vi "test TCX read (installed 71).vi"() -> ()   [LabVIEW 2011] (continued)
9</AltitudeMeters><DistanceMeters>17425.164</DistanceMeters><Cadence>84</Cadence><Extensions><TPX xmlns=\"http://www.garmin.com/xmlschemas/ActivityExtension/v2\"><Watts>247</Watts></TPX></Extensions></Trackpoint><Trackpoint><Time>2008-03-03T23:16:37Z</Time><Position><LatitudeDegrees>35.875664</LatitudeDegrees><LongitudeDegrees>-78.918461</LongitudeDegrees></Position><AltitudeMeters>60.220</AltitudeMeters><DistanceMeters>17434.398</DistanceMeters><Cadence>84</Cadence><Extensions><TPX xmlns=\"http://www.garmin.com/xmlschemas/ActivityExtension/v2\"><Watts>257</Watts></TPX></Extensions></Trackpoint><Trackpoint><Time>2008-03-03T23:16:38Z</Time><Position><LatitudeDegrees>35.875658</LatitudeDegrees><LongitudeDegrees>-78.918560</LongitudeDegrees></Position><AltitudeMeters>60.220</AltitudeMeters><DistanceMeters>17443.352</DistanceMeters><Cadence>83</Cadence><Extensions><TPX xmlns=\"http://www.garmin.com/xmlschemas/ActivityExtension/v2\"><Watts>228</Watts></TPX></Extensions></Trackpoint><Trackpoint><Time>2008-03-03T23:16:39Z</Time><Position><LatitudeDegrees>35.875651</LatitudeDegrees><LongitudeDegrees>-78.918658</LongitudeDegrees></Position><AltitudeMeters>60.220</AltitudeMeters><DistanceMeters>17452.232</DistanceMeters><Cadence>83</Cadence><Extensions><TPX xmlns=\"http://www.garmin.com/xmlschemas/ActivityExtension/v2\"><Watts>229</Watts></TPX></Extensions></Trackpoint><Trackpoint><Time>2008-03-03T23:16:40Z</Time><Position><LatitudeDegrees>35.875641</LatitudeDegrees><LongitudeDegrees>-78.918756</LongitudeDegrees></Position><AltitudeMeters>60.220</AltitudeMeters><DistanceMeters>17461.098</DistanceMeters><Cadence>81</Cadence><Extensions><TPX xmlns=\"http://www.garmin.com/xmlschemas/ActivityExtension/v2\"><Watts>206</Watts></TPX></Extensions></Trackpoint><Trackpoint><Time>2008-03-03T23:16:41Z</Time><Position><LatitudeDegrees>35.875632</LatitudeDegrees><LongitudeDegrees>-78.918851</LongitudeDegrees></Position><AltitudeMeters>60.220</AltitudeMeters><DistanceMeters>17469.729</DistanceMeters><Cadence>80</Cadence><Extensions><TPX xmlns=\"http://www.garmin.com/xmlschemas/ActivityExtension/v2\"><Watts>194</Watts></TPX></Extensions></Trackpoint><Trackpoint><Time>2008-03-03T23:16:42Z</Time><Position><LatitudeDegrees>35.875624</LatitudeDegrees><LongitudeDegrees>-78.918945</LongitudeDegrees></Position><AltitudeMeters>60.700</AltitudeMeters><DistanceMeters>17478.252</DistanceMeters><Cadence>77</Cadence><Extensions><TPX xmlns=\"http://www.garmin.com/xmlschemas/ActivityExtension/v2\"><Watts>145</Watts></TPX></Extensions></Trackpoint><Trackpoint><Time>2008-03-03T23:16:43Z</Time><Position><LatitudeDegrees>35.875617</LatitudeDegrees><LongitudeDegrees>-78.919037</LongitudeDegrees></Position><AltitudeMeters>60.220</AltitudeMeters><DistanceMeters>17486.607</DistanceMeters><Cadence>76</Cadence><Extensions><TPX xmlns=\"http://www.garmin.com/xmlschemas/ActivityExtension/v2\"><Watts>140</Watts></TPX></Extensions></Trackpoint><Trackpoint><Time>2008-03-03T23:16:44Z</Time><Position><LatitudeDegrees>35.875609</LatitudeDegrees><LongitudeDegrees>-78.919127</LongitudeDegrees></Position><AltitudeMeters>61.181</AltitudeMeters><DistanceMeters>17494.744</DistanceMeters><Cadence>74</Cadence><Extensions><TPX xmlns=\"http://www.garmin.com/xmlschemas/ActivityExtension/v2\"><Watts>140</Watts></TPX></Extensions></Trackpoint><Trackpoint><Time>2008-03-03T23:16:45Z</Time><Position><LatitudeDegrees>35.875602</LatitudeDegrees><LongitudeDegrees>-78.919214</LongitudeDegrees></Position><AltitudeMeters>61.181</AltitudeMeters><DistanceMeters>17502.676</DistanceMeters><Cadence>73</Cadence><Extensions><TPX xmlns=\"http://www.garmin.com/xmlschemas/ActivityExtension/v2\"><Watts>144</Watts></TPX></Extensions></Trackpoint><Trackpoint><Time>2008-03-03T23:16:46Z</Time><Position><LatitudeDegrees>35.875596</LatitudeDegrees><LongitudeDegrees>-78.919299</LongitudeDegrees></Position><AltitudeMeters>61.662</AltitudeMeters><DistanceMeters>17510.342</DistanceMeters><Cadence>71</Cadence><Extensions><TPX xmlns=\"http://www.garmin.com/xmlschemas/ActivityExtension/v2\"><Watts>160</Watts></TPX></Extensions></Trackpoint><Trackpoint><Time>2008-03-03T23:16:47Z</Time><Position><LatitudeDegrees>35.875590</LatitudeDegrees><LongitudeDegrees>-78.919382</LongitudeDegrees></Position><AltitudeMeters>61.181</AltitudeMeters><DistanceMeters>17517.861</DistanceMeters><Cadence>68</Cadence><Extensions><TPX xmlns=\"http://www.garmin.com/xmlschemas/ActivityExtension/v2\"><Watts>179</Watts></TPX></Extensions></Trackpoint><Trackpoint><Time>2008-03-03T23:16:48Z</Time><Position><LatitudeDegrees>35.875584</LatitudeDegrees><LongitudeDegrees>-78.919463</LongitudeDegrees></Position><AltitudeMeters>61.662</AltitudeMeters><DistanceMeters>17525.182</DistanceMeters><Cadence>67</Cadence><Extensions><TPX xmlns=\"http://www.garmin.com/xmlschemas/ActivityExtension/v2\"><Watts>190</Watts></TPX></Extensions></Trackpoint><Trackpoint><Time>2008-03-03T23:16:49Z</Time><Position><LatitudeDegrees>35.875578</LatitudeDegrees><LongitudeDegrees>-78.919542</LongitudeDegrees></Position><AltitudeMeters>61.662</AltitudeMeters><DistanceMeters>17532.338</DistanceMeters><Cadence>67</Cadence><Extensions><TPX xmlns=\"http://www.garmin.com/xmlschemas/ActivityExtension/v2\"><Watts>189</Watts></TPX></Extensions></Trackpoint><Trackpoint><Time>2008-03-03T23:16:50Z</Time><Position><LatitudeDegrees>35.875573</LatitudeDegrees><LongitudeDegrees>-78.919619</LongitudeDegrees></Position><AltitudeMeters>62.142</AltitudeMeters><DistanceMeters>17539.316</DistanceMeters><Cadence>65</Cadence><Extensions><TPX xmlns=\"http://www.garmin.com/xmlschemas/ActivityExtension/v2\"><Watts>213</Watts></TPX></Extensions></Trackpoint><Trackpoint><Time>2008-03-03T23:16:51Z</Time><Position><LatitudeDegrees>35.875567</LatitudeDegrees><LongitudeDegrees>-78.919694</LongitudeDegrees></Position><AltitudeMeters>62.142</AltitudeMeters><DistanceMeters>17546.102</DistanceMeters><Cadence>65</Cadence><Extensions><TPX xmlns=\"http://www.garmin.com/xmlschemas/ActivityExtension/v2\"><Watts>212</Watts></TPX></Extensions></Trackpoint><Trackpoint><Time>2008-03-03T23:16:52Z</Time><Position><LatitudeDegrees>35.875561</LatitudeDegrees><LongitudeDegrees>-78.919766</LongitudeDegrees></Position><AltitudeMeters>62.623</AltitudeMeters><DistanceMeters>17552.578</DistanceMeters><Cadence>67</Cadence><Extensions><TPX xmlns=\"http://www.garmin.com/xmlschemas/ActivityExtension/v2\"><Watts>211</Watts></TPX></Extensions></Trackpoint><Trackpoint><Time>2008-03-03T23:16:53Z</Time><Position><LatitudeDegrees>35.875555</LatitudeDegrees><LongitudeDegrees>-78.919835</LongitudeDegrees></Position><AltitudeMeters>62.623</AltitudeMeters><DistanceMeters>17558.822</DistanceMeters><Cadence>64</Cadence><Extensions><TPX xmlns=\"http://www.garmin.com/xmlschemas/ActivityExtension/v2\"><Watts>225</Watts></TPX></Extensions></Trackpoint><Trackpoint><Time>2008-03-03T23:16:54Z</Time><Position><LatitudeDegrees>35.875549</LatitudeDegrees><LongitudeDegrees>-78.919905</LongitudeDegrees></Position><AltitudeMeters>62.623</AltitudeMeters><DistanceMeters>17565.227</DistanceMeters><Cadence>66</Cadence><Extensions><TPX xmlns=\"http://www.garmin.com/xmlschemas/ActivityExtension/v2\"><Watts>266</Watts></TPX></Extensions></Trackpoint><Trackpoint><Time>2008-03-03T23:16:55Z</Time><Position><LatitudeDegrees>35.875535</LatitudeDegrees><LongitudeDegrees>-78.919978</LongitudeDegrees></Position><AltitudeMeters>63.104</AltitudeMeters><DistanceMeters>17571.996</DistanceMeters><Cadence>68</Cadence><Extensions><TPX xmlns=\"http://www.garmin.com/xmlschemas/ActivityExtension/v2\"><Watts>407</Watts></TPX></Extensions></Trackpoint><Trackpoint><Time>2008-03-03T23:16:56Z</Time><Position><LatitudeDegrees>35.875527</LatitudeDegrees><LongitudeDegrees>-78.920052</LongitudeDegrees></Position><AltitudeMeters>63.104</AltitudeMeters><DistanceMeters>17578.701</DistanceMeters><Cadence>71</Cadence><Extensions><TPX xmlns=\"http://www.garmin.com/xmlschemas/ActivityExtension/v2\"><Watts>440</Watts></TPX></Extensions></Trackpoint><Trackpoint><Time>2008-03-03T23:16:57Z</Time><Position><LatitudeDegrees>35.875524</LatitudeDegrees><LongitudeDegrees>-78.920126</LongitudeDegrees></Position><AltitudeMeters>63.584</AltitudeMeters><DistanceMeters>17585.479</DistanceMeters><Cadence>73</Cadence><Extensions><TPX xmlns=\"http://www.garmin.com/xmlschemas/ActivityExtension/v2\"><Watts>527</Watts></TPX></Extensions></Trackpoint><Trackpoint><Time>2008-03-03T23:16:58Z</Time><Position><LatitudeDegrees>35.875522</LatitudeDegrees><LongitudeDegrees>-78.920204</LongitudeDegrees></Position><AltitudeMeters>63.584</AltitudeMeters><DistanceMeters>17592.449</DistanceMeters><Cadence>74</Cadence><Extensions><TPX xmlns=\"http://www.garmin.com/xmlschemas/ActivityExtension/v2\"><Watts>618</Watts></TPX></Extensions></Trackpoint><Trackpoint><Time>2008-03-03T23:16:59Z</Time><Position><LatitudeDegrees>35.875519</LatitudeDegrees><LongitudeDegrees>-78.920284</LongitudeDegrees></Position><AltitudeMeters>64.065</AltitudeMeters><DistanceMeters>17599.703</DistanceMeters><Cadence>76</Cadence><Extensions><TPX xmlns=\"http://www.garmin.com/xmlschemas/ActivityExtension/v2\"><Watts>615</Watts></TPX></Extensions></Trackpoint><Trackpoint><Time>2008-03-03T23:17:00Z</Time><Position><LatitudeDegrees>35.875519</LatitudeDegrees><LongitudeDegrees>-78.920364</LongitudeDegrees></Position><AltitudeMeters>64.546</AltitudeMeters><DistanceMeters>17607.000</DistanceMeters><Cadence>76</Cadence><Extensions><TPX xmlns=\"http://www.garmin.com/xmlschemas/ActivityExtension/v2\"><Watts>600</Watts></TPX></Extensions></Trackpoint><Trackpoint><Time>2008-03-03T23:17:01Z</Time><Position><LatitudeDegrees>35.875518</LatitudeDegrees><LongitudeDegrees>-78.920446</LongitudeDegrees></Position><AltitudeMeters>65.507</AltitudeMeters><DistanceMeters>17614.344</DistanceMeters><Cadence>76</Cadence><Extensions><TPX xmlns=\"http://www.garmin.com/xmlschemas/ActivityExtension/v2\"><Watts>605</Watts></TPX></Extensions></Trackpoint><Trackpoint><Time>2008-03-03T23:17:02Z</Time><Position><LatitudeDegrees>35.875515</LatitudeDegrees><LongitudeDegrees>-78.920525</LongitudeDegrees></Position><AltitudeMeters>65.988</AltitudeMeters><DistanceMeters>17621.482</DistanceMeters><Cadence>73</Cadence><Extensions><TPX xmlns=\"http://www.garmin.com/xmlschemas/ActivityExtension/v2\"><Watts>509</Watts></TPX></Extensions></Trackpoint><Trackpoint><Time>2008-03-03T23:17:03Z</Time><Position><LatitudeDegrees>35.875514</LatitudeDegrees><LongitudeDegrees>-78.920601</LongitudeDegrees></Position><AltitudeMeters>66.468</AltitudeMeters><DistanceMeters>17628.330</DistanceMeters><Cadence>72</Cadence><Extensions><TPX xmlns=\"http://www.garmin.com/xmlschemas/ActivityExtension/v2\"><Watts>498</Watts></TPX></Extensions></Trackpoint><Trackpoint><Time>2008-03-03T23:17:04Z</Time><Position><LatitudeDegrees>35.875514</LatitudeDegrees><LongitudeDegrees>-78.920677</LongitudeDegrees></Position><AltitudeMeters>66.468</AltitudeMeters><DistanceMeters>17635.150</DistanceMeters><Cadence>71</Cadence><Extensions><TPX xmlns=\"http://www.garmin.com/xmlschemas/ActivityExtension/v2\"><Watts>409</Watts></TPX></Extensions></Trackpoint><Trackpoint><Time>2008-03-03T23:17:05Z</Time><Position><LatitudeDegrees>35.875514</LatitudeDegrees><LongitudeDegrees>-78.920753</LongitudeDegrees></Position><AltitudeMeters>66.468</AltitudeMeters><DistanceMeters>17642.037</DistanceMeters><Cadence>72</Cadence><Extensions><TPX xmlns=\"http://www.garmin.com/xmlschemas/ActivityExtension/v2\"><Watts>369</Watts></TPX></Extensions></Trackpoint><Trackpoint><Time>2008-03-03T23:17:06Z</Time><Position><LatitudeDegrees>35.875510</LatitudeDegrees><LongitudeDegrees>-78.920830</LongitudeDegrees></Position><AltitudeMeters>66.949</AltitudeMeters><DistanceMeters>17649.055</DistanceMeters><Cadence>73</Cadence><Extensions><TPX xmlns=\"http://www.garmin.com/xmlschemas/ActivityExtension/v2\"><Watts>334</Watts></TPX></Extensions></Trackpoint><Trackpoint><Time>2008-03-03T23:17:07Z</Time><Position><LatitudeDegrees>35.875506</LatitudeDegrees><LongitudeDegrees>-78.920910</LongitudeDegrees></Position><AltitudeMeters>67.430</AltitudeMeters><DistanceMeters>17656.324</DistanceMeters><Cadence>75</Cadence><Extensions><TPX xmlns=\"http://www.garmin.com/xmlschemas/ActivityExtension/v2\"><Watts>331</Watts></TPX></Extensions></Trackpoint><Trackpoint><Time>2008-03-03T23:17:08Z</Time><Position><LatitudeDegrees>35.875502</LatitudeDegrees><LongitudeDegrees>-78.920993</LongitudeDegrees></Position><AltitudeMeters>67.910</AltitudeMeters><DistanceMeters>17663.768</DistanceMeters><Cadence>79</Cadence><Extensions><TPX xmlns=\"http://www.garmin.com/xmlschemas/ActivityExtension/v2\"><Watts>322</Watts></TPX></Extensions></Trackpoint><Trackpoint><Time>2008-03-03T23:17:09Z</Time><Position><LatitudeDegrees>35.875499</LatitudeDegrees><LongitudeDegrees>-78.921077</LongitudeDegrees></Position><AltitudeMeters>67.430</AltitudeMeters><DistanceMeters>17671.379</DistanceMeters><Cadence>78</Cadence><Extensions><TPX xmlns=\"http://www.garmin.com/xmlschemas/ActivityExtension/v2\"><Watts>318</Watts></TPX></Extensions></Trackpoint><Trackpoint><Time>2008-03-03T23:17:10Z</Time><Position><LatitudeDegrees>35.875497</LatitudeDegrees><LongitudeDegrees>-78.921161</LongitudeDegrees></Position><AltitudeMeters>67.430</AltitudeMeters><DistanceMeters>17679.006</DistanceMeters><Cadence>78</Cadence><Extensions><TPX xmlns=\"http://www.garmin.com/xmlschemas/ActivityExtension/v2\"><Watts>224</Watts></TPX></Extensions></Trackpoint><Trackpoint><Time>2008-03-03T23:17:11Z</Time><Position><LatitudeDegrees>35.875497</LatitudeDegrees><LongitudeDegrees>-78.921246</LongitudeDegrees></Position><AltitudeMeters>67.430</AltitudeMeters><DistanceMeters>17686.682</DistanceMeters><Cadence>79</Cadence><Extensions><TPX xmlns=\"http://www.garmin.com/xmlschemas/ActivityExtension/v2\"><Watts>133</Watts></TPX></Extensions></Trackpoint><Trackpoint><Time>2008-03-03T23:17:12Z</Time><Position><LatitudeDegrees>35.875498</LatitudeDegrees><LongitudeDegrees>-78.921332</LongitudeDegrees></Position><AltitudeMeters>67.910</AltitudeMeters><DistanceMeters>17694.391</DistanceMeters><Cadence>79</Cadence><Extensions><TPX xmlns=\"http://www.garmin.com/xmlschemas/ActivityExtension/v2\"><Watts>116</Watts></TPX></Extensions></Trackpoint><Trackpoint><Time>2008-03-03T23:17:13Z</Time><Position><LatitudeDegrees>35.875497</LatitudeDegrees><LongitudeDegrees>-78.921417</LongitudeDegrees></Position><AltitudeMeters>67.910</AltitudeMeters><DistanceMeters>17702.156</DistanceMeters><Cadence>79</Cadence><Extensions><TPX xmlns=\"http://www.garmin.com/xmlschemas/ActivityExtension/v2\"><Watts>105</Watts></TPX></Extensions></Trackpoint><Trackpoint><Time>2008-03-03T23:17:14Z</Time><Position><LatitudeDegrees>35.875496</LatitudeDegrees><LongitudeDegrees>-78.921503</LongitudeDegrees></Position><AltitudeMeters>67.910</AltitudeMeters><DistanceMeters>17709.824</DistanceMeters><Cadence>79</Cadence><Extensions><TPX xmlns=\"http://www.garmin.com/xmlschemas/ActivityExtension/v2\"><Watts>101</Watts></TPX></Extensions></Trackpoint><Trackpoint><Time>2008-03-03T23:17:15Z</Time><Position><LatitudeDegrees>35.875492</LatitudeDegrees><LongitudeDegrees>-78.921586</LongitudeDegrees></Position><AltitudeMeters>67.910</AltitudeMeters><DistanceMeters>17717.307</DistanceMeters><Cadence>77</Cadence><Extensions><TPX xmlns=\"http://www.garmin.com/xmlschemas/ActivityExtension/v2\"><Watts>104</Watts></TPX></Extensions></Trackpoint><Trackpoint><Time>2008-03-03T23:17:16Z</Time><Position><LatitudeDegrees>35.875488</LatitudeDegrees><LongitudeDegrees>-78.921667</LongitudeDegrees></Position><AltitudeMeters>67.910</AltitudeMeters><DistanceMeters>17724.688</DistanceMeters><Cadence>77</Cadence><Extensions><TPX xmlns=\"http://www.garmin.com/xmlschemas/ActivityExtension/v2\"><Watts>103</Watts></TPX></Extensions></Trackpoint><Trackpoint><Time>2008-03-03T23:17:17Z</Time><Position><LatitudeDegrees>35.875483</LatitudeDegrees><LongitudeDegrees>-78.921747</LongitudeDegrees></Position><AltitudeMeters>67.910</AltitudeMeters><DistanceMeters>17731.865</DistanceMeters><Cadence>73</Cadence><Extensions><TPX xmlns=\"http://www.garmin.com/xmlschemas/ActivityExtension/v2\"><Watts>125</Watts></TPX></Extensions></Trackpoint><Trackpoint><Time>2008-03-03T23:17:18Z</Time><Position><LatitudeDegrees>35.875477</LatitudeDegrees><LongitudeDegrees>-78.921826</LongitudeDegrees></Position><AltitudeMeters>67.910</AltitudeMeters><DistanceMeters>17739.020</DistanceMeters><Cadence>75</Cadence><Extensions><TPX xmlns=\"http://www.garmin.com/xmlschemas/ActivityExtension/v2\"><Watts>187</Watts></TPX></Extensions></Trackpoint><Trackpoint><Time>2008-03-03T23:17:19Z</Time><Position><LatitudeDegrees>35.875471</LatitudeDegrees><LongitudeDegrees>-78.921905</LongitudeDegrees></Position><AltitudeMeters>68.391</AltitudeMeters><DistanceMeters>17746.203</DistanceMeters><Cadence>75</Cadence><Extensions><TPX xmlns=\"http://www.garmin.com/xmlschemas/ActivityExtension/v2\"><Watts>304</Watts></TPX></Extensions></Trackpoint><Trackpoint><Time>2008-03-03T23:17:20Z</Time><Position><LatitudeDegrees>35.875465</LatitudeDegrees><LongitudeDegrees>-78.921982</LongitudeDegrees></Position><AltitudeMeters>68.872</AltitudeMeters><DistanceMeters>17753.166</DistanceMeters><Cadence>73</Cadence><Extensions><TPX xmlns=\"http://www.garmin.com/xmlschemas/ActivityExtension/v2\"><Watts>365</Watts></TPX></Extensions></Trackpoint><Trackpoint><Time>2008-03-03T23:17:21Z</Time><Position><LatitudeDegrees>35.875460</LatitudeDegrees><LongitudeDegrees>-78.922058</LongitudeDegrees></Position><AltitudeMeters>68.872</AltitudeMeters><DistanceMeters>17760.088</DistanceMeters><Cadence>73</Cadence><Extensions><TPX xmlns=\"http://www.garmin.com/xmlschemas/ActivityExtension/v2\"><Watts>361</Watts></TPX></Extensions></Trackpoint><Trackpoint><Time>2008-03-03T23:17:22Z</Time><Position><LatitudeDegrees>35.875456</LatitudeDegrees><LongitudeDegrees>-78.922133</LongitudeDegrees></Position><AltitudeMeters>69.352</AltitudeMeters><DistanceMeters>17766.865</DistanceMeters><Cadence>70</Cadence><Extensions><TPX xmlns=\"http://www.garmin.com/xmlschemas/ActivityExtension/v2\"><Watts>317</Watts></TPX></Extensions></Trackpoint><Trackpoint><Time>2008-03-03T23:17:23Z</Time><Position><LatitudeDegrees>35.875451</LatitudeDegrees><LongitudeDegrees>-78.922207</LongitudeDegrees></Position><AltitudeMeters>69.833</AltitudeMeters><DistanceMeters>17773.584</DistanceMeters><Cadence>70</Cadence><Extensions><TPX xmlns=\"http://www.garmin.com/xmlschemas/ActivityExtension/v2\"><Watts>340</Watts></TPX></Extensions></Trackpoint><Trackpoint><Time>2008-03-03T23:17:24Z</Time><Position><LatitudeDegrees>35.875446</LatitudeDegrees><LongitudeDegrees>-78.922283</LongitudeDegrees></Position><AltitudeMeters>69.833</AltitudeMeters><DistanceMeters>17780.492</DistanceMeters><Cadence>75</Cadence><Extensions><TPX xmlns=\"http://www.garmin.com/xmlschemas/ActivityExtension/v2\"><Watts>332</Watts></TPX></Extensions></Trackpoint><Trackpoint><Time>2008-03-03T23:17:25Z</Time><Position><LatitudeDegrees>35.875445</LatitudeDegrees><LongitudeDegrees>-78.922363</LongitudeDegrees></Position><AltitudeMeters>70.313</AltitudeMeters><DistanceMeters>17787.660</DistanceMeters><Cadence>73</Cadence><Extensions><TPX xmlns=\"http://www.garmin.com/xmlschemas/ActivityExtension/v2\"><Watts>305</Watts></TPX></Extensions></Trackpoint><Trackpoint><Time>2008-03-03T23:17:26Z</Time><Position><LatitudeDegrees>35.875444</LatitudeDegrees><LongitudeDegrees>-78.922441</LongitudeDegrees></Position><AltitudeMeters>70.313</AltitudeMeters><DistanceMeters>17794.773</DistanceMeters><Cadence>73</Cadence><Extensions><TPX xmlns=\"http://www.garmin.com/xmlschemas/ActivityExtension/v2\"><Watts>224</Watts></TPX></Extensions></Trackpoint><Trackpoint><Time>2008-03-03T23:17:27Z</Time><Position><LatitudeDegrees>35.875442</LatitudeDegrees><LongitudeDegrees>-78.922520</LongitudeDegrees></Position><AltitudeMeters>70.313</AltitudeMeters><DistanceMeters>17801.924</DistanceMeters><Cadence>74</Cadence><Extensions><TPX xmlns=\"http://www.garmin.com/xmlschemas/ActivityExtension/v2\"><Watts>148</Watts></TPX></Extensions></Trackpoint><Trackpoint><Time>2008-03-03T23:17:28Z</Time><Position><LatitudeDegrees>35.875442</LatitudeDegrees><LongitudeDegrees>-78.922601</LongitudeDegrees></Position><AltitudeMeters>70.313</AltitudeMeters><DistanceMeters>17809.150</DistanceMeters><Cadence>74</Cadence><Extensions><TPX xmlns=\"http://www.garmin.com/xmlschemas/ActivityExtension/v2\"><Watts>122</Watts></TPX></Extensions></Trackpoint><Trackpoint><Time>2008-03-03T23:17:29Z</Time><Position><LatitudeDegrees>35.875442</LatitudeDegrees><LongitudeDegrees>-78.922683</LongitudeDegrees></Position><AltitudeMeters>70.794</AltitudeMeters><DistanceMeters>17816.596</DistanceMeters><Cadence>77</Cadence><Extensions><TPX xmlns=\"http://www.garmin.com/xmlschemas/ActivityExtension/v2\"><Watts>92</Watts></TPX></Extensions></Trackpoint><Trackpoint><Time>2008-03-03T23:17:30Z</Time><Position><LatitudeDegrees>35.875443</LatitudeDegrees><LongitudeDegrees>-78.922767</LongitudeDegrees></Position><AltitudeMeters>69.833</AltitudeMeters><DistanceMeters>17824.229</DistanceMeters><Cadence>79</Cadence><Extensions><TPX xmlns=\"http://www.garmin.com/xmlschemas/ActivityExtension/v2\"><Watts>79</Watts></TPX></Extensions></Trackpoint><Trackpoint><Time>2008-03-03T23:17:31Z</Time><Position><LatitudeDegrees>35.875442</LatitudeDegrees><LongitudeDegrees>-78.922856</LongitudeDegrees></Position><AltitudeMeters>69.833</AltitudeMeters><DistanceMeters>17832.281</DistanceMeters><Cadence>68</Cadence><Extensions><TPX xmlns=\"http://www.garmin.com/xmlschemas/ActivityExtension/v2\"><Watts>70</Watts></TPX></Extensions></Trackpoint><Trackpoint><Time>2008-03-03T23:17:32Z</Time><Position><LatitudeDegrees>35.875442</LatitudeDegrees><LongitudeDegrees>-78.922951</LongitudeDegrees></Position><AltitudeMeters>69.352</AltitudeMeters><DistanceMeters>17840.867</DistanceMeters><Cadence>69</Cadence><Extensions><TPX xmlns=\"http://www.garmin.com/xmlschemas/ActivityExtension/v2\"><Watts>69</Watts></TPX></Extensions></Trackpoint><Trackpoint><Time>2008-03-03T23:17:33Z</Time><Position><LatitudeDegrees>35.875442</LatitudeDegrees><LongitudeDegrees>-78.923052</LongitudeDegrees></Position><AltitudeMeters>69.352</AltitudeMeters><DistanceMeters>17850.025</DistanceMeters><Cadence>73</Cadence><Extensions><TPX xmlns=\"http://www.garmin.com/xmlschemas/ActivityExtension/v2\"><Watts>69</Watts></TPX></Extensions></Trackpoint><Trackpoint><Time>2008-03-03T23:17:34Z</Time><Position><LatitudeDegrees>35.875441</LatitudeDegrees><LongitudeDegrees>-78.923158</LongitudeDegrees></Position><AltitudeMeters>68.872</AltitudeMeters><DistanceMeters>17859.643</DistanceMeters><Cadence>78</Cadence><Extensions><TPX xmlns=\"http://www.garmin.com/xmlschemas/ActivityExtension/v2\"><Watts>67</Watts></TPX></Extensions></Trackpoint><Trackpoint><Time>2008-03-03T23:17:35Z</Time><Position><LatitudeDegrees>35.875440</LatitudeDegrees><LongitudeDegrees>-78.923269</LongitudeDegrees></Position><AltitudeMeters>68.391</AltitudeMeters><DistanceMeters>17869.717</DistanceMeters><Cadence>82</Cadence><Extensions><TPX xmlns=\"http://www.garmin.com/xmlschemas/ActivityExtension/v2\"><Watts>66</Watts></TPX></Extensions></Trackpoint><Trackpoint><Time>2008-03-03T23:17:36Z</Time><Position><LatitudeDegrees>35.875439</LatitudeDegrees><LongitudeDegrees>-78.923384</LongitudeDegrees></Position><AltitudeMeters>67.910</AltitudeMeters><DistanceMeters>17880.117</DistanceMeters><Cadence>84</Cadence><Extensions><TPX xmlns=\"http://www.garmin.com/xmlschemas/ActivityExtension/v2\"><Watts>65</Watts></TPX></Extensions></Trackpoint><Trackpoint><Time>2008-03-03T23:17:37Z</Time><Position><LatitudeDegrees>35.875439</LatitudeDegrees><LongitudeDegrees>-78.923501</LongitudeDegrees></Position><AltitudeMeters>67.910</AltitudeMeters><DistanceMeters>17890.664</DistanceMeters><Cadence>86</Cadence><Extensions><TPX xmlns=\"http://www.garmin.com/xmlschemas/ActivityExtension/v2\"><Watts>67</Watts></TPX></Extensions></Trackpoint><Trackpoint><Time>2008-03-03T23:17:38Z</Time><Position><LatitudeDegrees>35.875439</LatitudeDegrees><LongitudeDegrees>-78.923620</LongitudeDegrees></Position><AltitudeMeters>67.430</AltitudeMeters><DistanceMeters>17901.379</DistanceMeters><Cadence>87</Cadence><Extensions><TPX xmlns=\"http://www.garmin.com/xmlschemas/ActivityExtension/v2\"><Watts>74</Watts></TPX></Extensions></Trackpoint><Trackpoint><Time>2008-03-03T23:17:39Z</Time><Position><LatitudeDegrees>35.875437</LatitudeDegrees><LongitudeDegrees>-78.923739</LongitudeDegrees></Position><AltitudeMeters>66.949</AltitudeMeters><DistanceMeters>17912.166</DistanceMeters><Cadence>88</Cadence><Extensions><TPX xmlns=\"http://www.garmin.com/xmlschemas/ActivityExtension/v2\"><Watts>82</Watts></TPX></Extensions></Trackpoint><Trackpoint><Time>2008-03-03T23:17:40Z</Time><Position><LatitudeDegrees>35.875435</LatitudeDegrees><LongitudeDegrees>-78.923858</LongitudeDegrees></Position><AltitudeMeters>66.468</AltitudeMeters><DistanceMeters>17922.941</DistanceMeters><Cadence>88</Cadence><Extensions><TPX xmlns=\"http://www.garmin.com/xmlschemas/ActivityExtension/v2\"><Watts>86</Watts></TPX></Extensions></Trackpoint><Trackpoint><Time>2008-03-03T23:17:41Z</Time><Position><LatitudeDegrees>35.875433</LatitudeDegrees><LongitudeDegrees>-78.923977</LongitudeDegrees></Position><AltitudeMeters>65.988</AltitudeMeters><DistanceMeters>17933.627</DistanceMeters><Cadence>87</Cadence><Extensions><TPX xmlns=\"http://www.garmin.com/xmlschemas/ActivityExtension/v2\"><Watts>89</Watts></TPX></Extensions></Trackpoint><Trackpoint><Time>2008-03-03T23:17:42Z</Time><Position><LatitudeDegrees>35.875433</LatitudeDegrees><LongitudeDegrees>-78.924094</LongitudeDegrees></Position><AltitudeMeters>65.988</AltitudeMeters><DistanceMeters>17944.260</DistanceMeters><Cadence>86</Cadence><Extensions><TPX xmlns=\"http://www.garmin.com/xmlschemas/ActivityExtension/v2\"><Watts>91</Watts></TPX></Extensions></Trackpoint><Trackpoint><Time>2008-03-03T23:17:43Z</Time><Position><LatitudeDegrees>35.875432</LatitudeDegrees><LongitudeDegrees>-78.924211</LongitudeDegrees></Position><AltitudeMeters>65.988</AltitudeMeters><DistanceMeters>17954.787</DistanceMeters><Cadence>85</Cadence><Extensions><TPX xmlns=\"http://www.garmin.com/xmlschemas/ActivityExtension/v2\"><Watts>98</Watts></TPX></Extensions></Trackpoint><Trackpoint><Time>2008-03-03T23:17:44Z</Time><Position><LatitudeDegrees>35.875431</LatitudeDegrees><LongitudeDegrees>-78.924328</LongitudeDegrees></Position><AltitudeMeters>65.988</AltitudeMeters><DistanceMeters>17965.385</DistanceMeters><Cadence>86</Cadence><Extensions><TPX xmlns=\"http://www.garmin.com/xmlschemas/ActivityExtension/v2\"><Watts>120</Watts></TPX></Extensions></Trackpoint><Trackpoint><Time>2008-03-03T23:17:45Z</Time><Position><LatitudeDegrees>35.875430</LatitudeDegrees><LongitudeDegrees>-78.924446</LongitudeDegrees></Position><AltitudeMeters>65.026</AltitudeMeters><DistanceMeters>17976.049</DistanceMeters><Cadence>87</Cadence><Extensions><TPX xmlns=\"http://www.garmin.com/xmlschemas/ActivityExtension/v2\"><Watts>153</Watts></TPX></Extensions></Trackpoint><Trackpoint><Time>2008-03-03T23:17:46Z</Time><Position><LatitudeDegrees>35.875429</LatitudeDegrees><LongitudeDegrees>-78.924565</LongitudeDegrees></Position><AltitudeMeters>65.507</AltitudeMeters><DistanceMeters>17986.748</DistanceMeters><Cadence>87</Cadence><Extensions><TPX xmlns=\"http://www.garmin.com/xmlschemas/ActivityExtension/v2\"><Watts>153</Watts></TPX></Extensions></Trackpoint><Trackpoint><Time>2008-03-03T23:17:47Z</Time><Position><LatitudeDegrees>35.875429</LatitudeDegrees><LongitudeDegrees>-78.924684</LongitudeDegrees></Position><AltitudeMeters>65.026</AltitudeMeters><DistanceMeters>17997.576</DistanceMeters><Cadence>87</Cadence><Extensions><TPX xmlns=\"http://www.garmin.com/xmlschemas/ActivityExtension/v2\"><Watts>135</Watts></TPX></Extensions></Trackpoint><Trackpoint><Time>2008-03-03T23:17:48Z</Time><Position><LatitudeDegrees>35.875428</LatitudeDegrees><LongitudeDegrees>-78.924804</LongitudeDegrees></Position><AltitudeMeters>65.026</AltitudeMeters><DistanceMeters>18008.354</DistanceMeters><Cadence>87</Cadence><Extensions><TPX xmlns=\"http://www.garmin.com/xmlschemas/ActivityExtension/v2\"><Watts>135</Watts></TPX></Extensions></Trackpoint><Trackpoint><Time>2008-03-03T23:17:49Z</Time><Position><LatitudeDegrees>35.875427</LatitudeDegrees><LongitudeDegrees>-78.924925</LongitudeDegrees></Position><AltitudeMeters>65.026</AltitudeMeters><DistanceMeters>18019.271</DistanceMeters><Cadence>89</Cadence><Extensions><TPX xmlns=\"http://www.garmin.com/xmlschemas/ActivityExtension/v2\"><Watts>104</Watts></TPX></Extensions></Trackpoint><Trackpoint><Time>2008-03-03T23:17:50Z</Time><Position><LatitudeDegrees>35.875426</LatitudeDegrees><LongitudeDegrees>-78.925047</LongitudeDegrees></Position><AltitudeMeters>64.065</AltitudeMeters><DistanceMeters>18030.314</DistanceMeters><Cadence>89</Cadence><Extensions><TPX xmlns=\"http://www.garmin.com/xmlschemas/ActivityExtension/v2\"><Watts>104</Watts></TPX></Extensions></Trackpoint><Trackpoint><Time>2008-03-03T23:17:51Z</Time><Position><LatitudeDegrees>35.875425</LatitudeDegrees><LongitudeDegrees>-78.925169</LongitudeDegrees></Position><AltitudeMeters>63.584</AltitudeMeters><DistanceMeters>18041.348</DistanceMeters><Cadence>90</Cadence><Extensions><TPX xmlns=\"http://www.garmin.com/xmlschemas/ActivityExtension/v2\"><Watts>84</Watts></TPX></Extensions></Trackpoint><Trackpoint><Time>2008-03-03T23:17:52Z</Time><Position><LatitudeDegrees>35.875424</LatitudeDegrees><LongitudeDegrees>-78.925291</LongitudeDegrees></Position><AltitudeMeters>64.065</AltitudeMeters><DistanceMeters>18052.355</DistanceMeters><Cadence>90</Cadence><Extensions><TPX xmlns=\"http://www.garmin.com/xmlschemas/ActivityExtension/v2\"><Watts>75</Watts></TPX></Extensions></Trackpoint><Trackpoint><Time>2008-03-03T23:17:53Z</Time><Position><LatitudeDegrees>35.875426</LatitudeDegrees><LongitudeDegrees>-78.925412</LongitudeDegrees></Position><AltitudeMeters>64.065</AltitudeMeters><DistanceMeters>18063.305</DistanceMeters><Cadence>90</Cadence><Extensions><TPX xmlns=\"http://www.garmin.com/xmlschemas/ActivityExtension/v2\"><Watts>76</Watts></TPX></Extensions></Trackpoint><Trackpoint><Time>2008-03-03T23:17:54Z</Time><Position><LatitudeDegrees>35.875427</LatitudeDegrees><LongitudeDegrees>-78.925533</LongitudeDegrees></Position><AltitudeMeters>64.065</AltitudeMeters><DistanceMeters>18074.193</DistanceMeters><Cadence>89</Cadence><Extensions><TPX xmlns=\"http://www.garmin.com/xmlschemas/ActivityExtension/v2\"><Watts>79</Watts></TPX></Extensions></Trackpoint><Trackpoint><Time>2008-03-03T23:17:55Z</Time><Position><LatitudeDegrees>35.875427</LatitudeDegrees><LongitudeDegrees>-78.925652</LongitudeDegrees></Position><AltitudeMeters>63.584</AltitudeMeters><DistanceMeters>18084.902</DistanceMeters><Cadence>88</Cadence><Extensions><TPX xmlns=\"http://www.garmin.com/xmlschemas/ActivityExtension/v2\"><Watts>88</Watts></TPX></Extensions></Trackpoint><Trackpoint><Time>2008-03-03T23:17:56Z</Time><Position><LatitudeDegrees>35.875428</LatitudeDegrees><LongitudeDegrees>-78.925770</LongitudeDegrees></Position><AltitudeMeters>64.065</AltitudeMeters><DistanceMeters>18095.518</DistanceMeters><Cadence>86</Cadence><Extensions><TPX xmlns=\"http://www.garmin.com/xmlschemas/ActivityExtension/v2\"><Watts>92</Watts></TPX></Extensions></Trackpoint><Trackpoint><Time>2008-03-03T23:17:57Z</Time><Position><LatitudeDegrees>35.875428</LatitudeDegrees><LongitudeDegrees>-78.925885</LongitudeDegrees></Position><AltitudeMeters>63.584</AltitudeMeters><DistanceMeters>18105.930</DistanceMeters><Cadence>85</Cadence><Extensions><TPX xmlns=\"http://www.garmin.com/xmlschemas/ActivityExtension/v2\"><Watts>100</Watts></TPX></Extensions></Trackpoint><Trackpoint><Time>2008-03-03T23:17:58Z</Time><Position><LatitudeDegrees>35.875428</LatitudeDegrees><LongitudeDegrees>-78.925998</LongitudeDegrees></Position><AltitudeMeters>63.584</AltitudeMeters><DistanceMeters>18116.090</DistanceMeters><Cadence>83</Cadence><Extensions><TPX xmlns=\"http://www.garmin.com/xmlschemas/ActivityExtension/v2\"><Watts>109</Watts></TPX></Extensions></Trackpoint><Trackpoint><Time>2008-03-03T23:17:59Z</Time><Position><LatitudeDegrees>35.875428</LatitudeDegrees><LongitudeDegrees>-78.926107</LongitudeDegrees></Position><AltitudeMeters>63.584</AltitudeMeters><DistanceMeters>18125.930</DistanceMeters><Cadence>80</Cadence><Extensions><TPX xmlns=\"http://www.garmin.com/xmlschemas/ActivityExtension/v2\"><Watts>110</Watts></TPX></Extensions></Trackpoint><Trackpoint><Time>2008-03-03T23:18:00Z</Time><Position><LatitudeDegrees>35.875431</LatitudeDegrees><LongitudeDegrees>-78.926211</LongitudeDegrees></Position><AltitudeMeters>64.065</AltitudeMeters><DistanceMeters>18135.336</DistanceMeters><Cadence>80</Cadence><Extensions><TPX xmlns=\"http://www.garmin.com/xmlschemas/ActivityExtension/v2\"><Watts>109</Watts></TPX></Extensions></Trackpoint><Trackpoint><Time>2008-03-03T23:18:01Z</Time><Position><LatitudeDegrees>35.875440</LatitudeDegrees><LongitudeDegrees>-78.926310</LongitudeDegrees></Position><AltitudeMeters>64.065</AltitudeMeters><DistanceMeters>18144.322</DistanceMeters><Cadence>70</Cadence><Extensions><TPX xmlns=\"http://www.garmin.com/xmlschemas/ActivityExtension/v2\"><Watts>113</Watts></TPX></Extensions></Trackpoint><Trackpoint><Time>2008-03-03T23:18:02Z</Time><Position><LatitudeDegrees>35.875449</LatitudeDegrees><LongitudeDegrees>-78.926403</LongitudeDegrees></Position><AltitudeMeters>64.546</AltitudeMeters><DistanceMeters>18152.730</DistanceMeters><Cadence>70</Cadence><Extensions><TPX xmlns=\"http://www.garmin.com/xmlschemas/ActivityExtension/v2\"><Watts>98</Watts></TPX></Extensions></Trackpoint><Trackpoint><Time>2008-03-03T23:18:03Z</Time><Position><LatitudeDegrees>35.875455</LatitudeDegrees><LongitudeDegrees>-78.926490</LongitudeDegrees></Position><AltitudeMeters>64.546</AltitudeMeters><DistanceMeters>18160.592</DistanceMeters><Cadence>76</Cadence><Extensions><TPX xmlns=\"http://www.garmin.com/xmlschemas/ActivityExtension/v2\"><Watts>114</Watts></TPX></Extensions></Trackpoint><Trackpoint><Time>2008-03-03T23:18:04Z</Time><Position><LatitudeDegrees>35.875462</LatitudeDegrees><LongitudeDegrees>-78.926573</LongitudeDegrees></Position><AltitudeMeters>64.546</AltitudeMeters><DistanceMeters>18168.061</DistanceMeters><Cadence>76</Cadence><Extensions><TPX xmlns=\"http://www.garmin.com/xmlschemas/ActivityExtension/v2\"><Watts>270</Watts></TPX></Extensions></Trackpoint><Trackpoint><Time>2008-03-03T23:18:05Z</Time><Position><LatitudeDegrees>35.875469</LatitudeDegrees><LongitudeDegrees>-78.926654</LongitudeDegrees></Position><AltitudeMeters>65.507</AltitudeMeters><DistanceMeters>18175.398</DistanceMeters><Cadence>76</Cadence><Extensions><TPX xmlns=\"http://www.garmin.com/xmlschemas/ActivityExtension/v2\"><Watts>274</Watts></TPX></Extensions></Trackpoint><Trackpoint><Time>2008-03-03T23:18:06Z</Time><Position><LatitudeDegrees>35.875477</LatitudeDegrees><LongitudeDegrees>-78.926734</LongitudeDegrees></Position><AltitudeMeters>65.507</AltitudeMeters><DistanceMeters>18182.648</DistanceMeters><Cadence>75</Cadence><Extensions><TPX xmlns=\"http://www.garmin.com/xmlschemas/ActivityExtension/v2\"><Watts>511</Watts></TPX></Extensions></Trackpoint><Trackpoint><Time>2008-03-03T23:18:07Z</Time><Position><LatitudeDegrees>35.875486</LatitudeDegrees><LongitudeDegrees>-78.926811</LongitudeDegrees></Position><AltitudeMeters>65.507</AltitudeMeters><DistanceMeters>18189.766</DistanceMeters><Cadence>75</Cadence><Extensions><TPX xmlns=\"http://www.garmin.com/xmlschemas/ActivityExtension/v2\"><Watts>509</Watts></TPX></Extensions></Trackpoint><Trackpoint><Time>2008-03-03T23:18:08Z</Time><Position><LatitudeDegrees>35.875494</LatitudeDegrees><LongitudeDegrees>-78.926887</LongitudeDegrees></Position><AltitudeMeters>66.468</AltitudeMeters><DistanceMeters>18196.645</DistanceMeters><Cadence>73</Cadence><Extensions><TPX xmlns=\"http://www.garmin.com/xmlschemas/ActivityExtension/v2\"><Watts>465</Watts></TPX></Extensions></Trackpoint><Trackpoint><Time>2008-03-03T23:18:09Z</Time><Position><LatitudeDegrees>35.875504</LatitudeDegrees><LongitudeDegrees>-78.926962</LongitudeDegrees></Position><AltitudeMeters>66.949</AltitudeMeters><DistanceMeters>18203.498</DistanceMeters><Cadence>72</Cadence><Extensions><TPX xmlns=\"http://www.garmin.com/xmlschemas/ActivityExtension/v2\"><Watts>418</Watts></TPX></Extensions></Trackpoint><Trackpoint><Time>2008-03-03T23:18:10Z</Time><Position><LatitudeDegrees>35.875512</LatitudeDegrees><LongitudeDegrees>-78.927036</LongitudeDegrees></Position><AltitudeMeters>67.430</AltitudeMeters><DistanceMeters>18210.244</DistanceMeters><Cadence>72</Cadence><Extensions><TPX xmlns=\"http://www.garmin.com/xmlschemas/ActivityExtension/v2\"><Watts>418</Watts></TPX></Extensions></Trackpoint><Trackpoint><Time>2008-03-03T23:18:11Z</Time><Position><LatitudeDegrees>35.875519</LatitudeDegrees><LongitudeDegrees>-78.927111</LongitudeDegrees></Position><AltitudeMeters>67.910</AltitudeMeters><DistanceMeters>18217.014</DistanceMeters><Cadence>71</Cadence><Extensions><TPX xmlns=\"http://www.garmin.com/xmlschemas/ActivityExtension/v2\"><Watts>411</Watts></TPX></Extensions></Trackpoint><Trackpoint><Time>2008-03-03T23:18:12Z</Time><Position><LatitudeDegrees>35.875527</LatitudeDegrees><LongitudeDegrees>-78.927186</LongitudeDegrees></Position><AltitudeMeters>67.910</AltitudeMeters><DistanceMeters>18223.904</DistanceMeters><Cadence>72</Cadence><Extensions><TPX xmlns=\"http://www.garmin.com/xmlschemas/ActivityExtension/v2\"><Watts>384</Watts></TPX></Extensions></Trackpoint><Trackpoint><Time>2008-03-03T23:18:13Z</Time><Position><LatitudeDegrees>35.875534</LatitudeDegrees><LongitudeDegrees>-78.927262</LongitudeDegrees></Position><AltitudeMeters>67.910</AltitudeMeters><DistanceMeters>18230.748</DistanceMeters><Cadence>71</Cadence><Extensions><TPX xmlns=\"http://www.garmin.com/xmlschemas/ActivityExtension/v2\"><Watts>301</Watts></TPX></Extensions></Trackpoint><Trackpoint><Time>2008-03-03T23:18:14Z</Time><Position><LatitudeDegrees>35.875540</LatitudeDegrees><LongitudeDegrees>-78.927337</LongitudeDegrees></Position><AltitudeMeters>67.910</AltitudeMeters><DistanceMeters>18237.568</DistanceMeters><Cadence>72</Cadence><Extensions><TPX xmlns=\"http://www.garmin.com/xmlschemas/ActivityExtension/v2\"><Watts>275</Watts></TPX></Extensions></Trackpoint><Trackpoint><Time>2008-03-03T23:18:15Z</Time><Position><LatitudeDegrees>35.875547</LatitudeDegrees><LongitudeDegrees>-78.927412</LongitudeDegrees></Position><AltitudeMeters>68.391</AltitudeMeters><DistanceMeters>18244.424</DistanceMeters><Cadence>72</Cadence><Extensions><TPX xmlns=\"http://www.garmin.com/xmlschemas/ActivityExtension/v2\"><Watts>243</Watts></TPX></Extensions></Trackpoint><Trackpoint><Time>2008-03-03T23:18:16Z</Time><Position><LatitudeDegrees>35.875554</LatitudeDegrees><LongitudeDegrees>-78.927489</LongitudeDegrees></Position><AltitudeMeters>68.872</AltitudeMeters><DistanceMeters>18251.369</DistanceMeters><Cadence>72</Cadence><Extensions><TPX xmlns=\"http://www.garmin.com/xmlschemas/ActivityExtension/v2\"><Watts>215</Watts></TPX></Extensions></Trackpoint><Trackpoint><Time>2008-03-03T23:18:17Z</Time><Position><LatitudeDegrees>35.875560</LatitudeDegrees><LongitudeDegrees>-78.927566</LongitudeDegrees></Position><AltitudeMeters>68.391</AltitudeMeters><DistanceMeters>18258.379</DistanceMeters><Cadence>72</Cadence><Extensions><TPX xmlns=\"http://www.garmin.com/xmlschemas/ActivityExtension/v2\"><Watts>216</Watts></TPX></Extensions></Trackpoint><Trackpoint><Time>2008-03-03T23:18:18Z</Time><Position><LatitudeDegrees>35.875565</LatitudeDegrees><LongitudeDegrees>-78.927643</LongitudeDegrees></Position><AltitudeMeters>68.391</AltitudeMeters><DistanceMeters>18265.371</DistanceMeters><Cadence>74</Cadence><Extensions><TPX xmlns=\"http://www.garmin.com/xmlschemas/ActivityExtension/v2\"><Watts>165</Watts></TPX></Extensions></Trackpoint><Trackpoint><Time>2008-03-03T2
